vi "Cowl.vi"() -> ()   [LabVIEW 2019]
uses:
  outputs.vi
panel:
  out "Numeric":dbl
  in  "Desired_State 3":string
  in  "Desired_State 2":string
  in  "Desired_State":string
  in  "Current_State":string
  in  "Boolean":bool
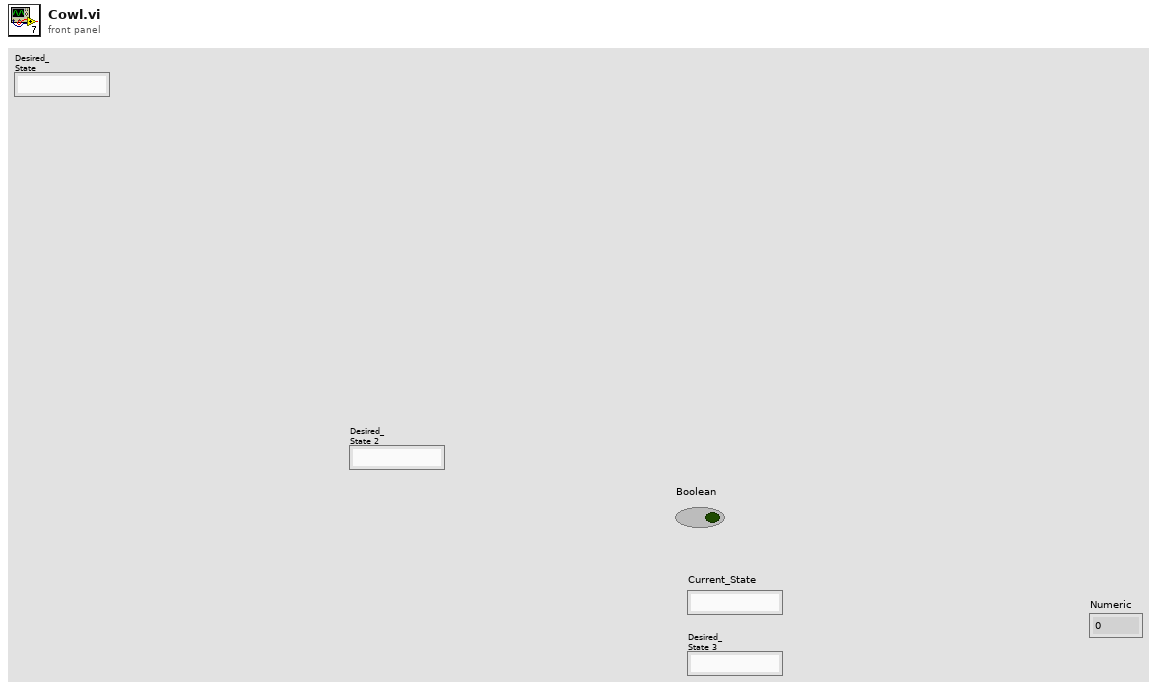
[diagram p1: front panel]
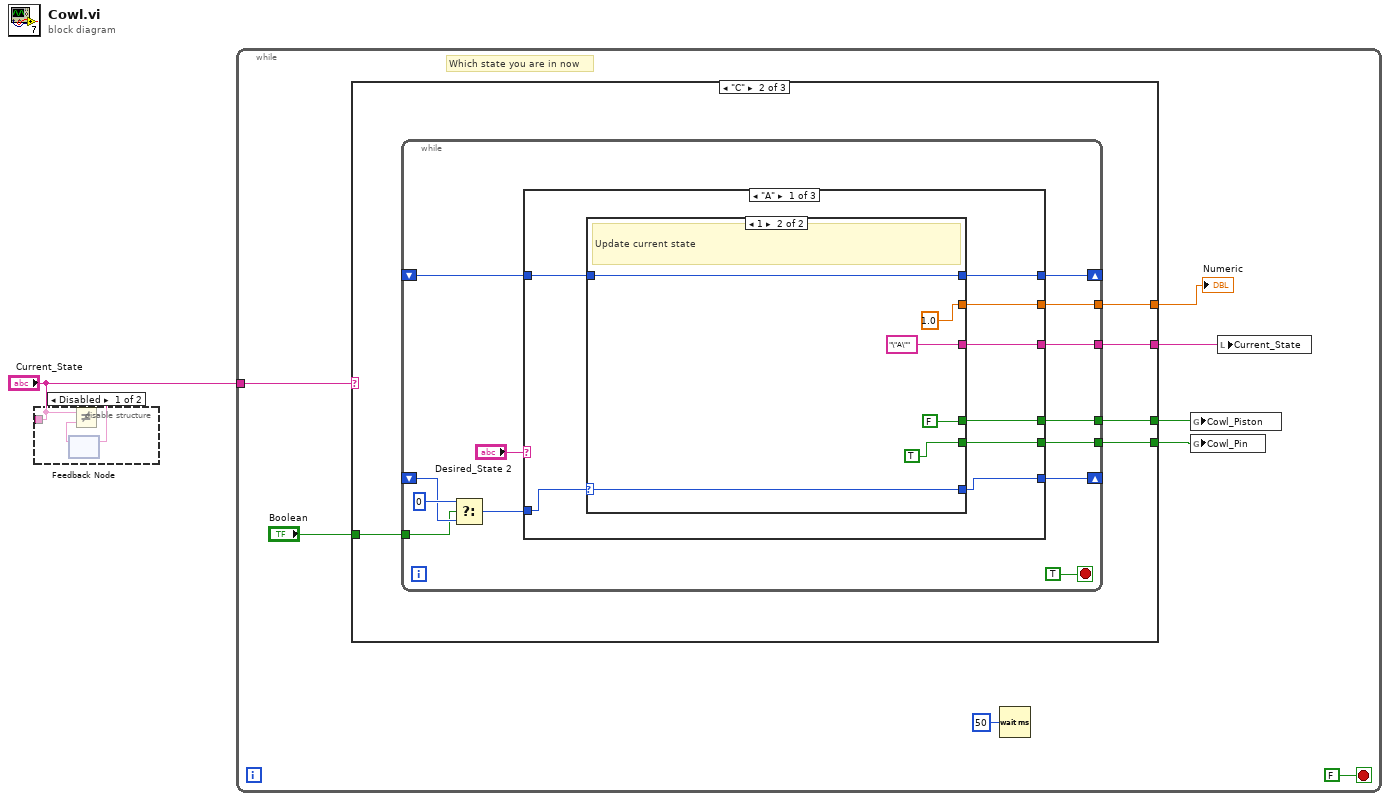
[diagram p0: block diagram]
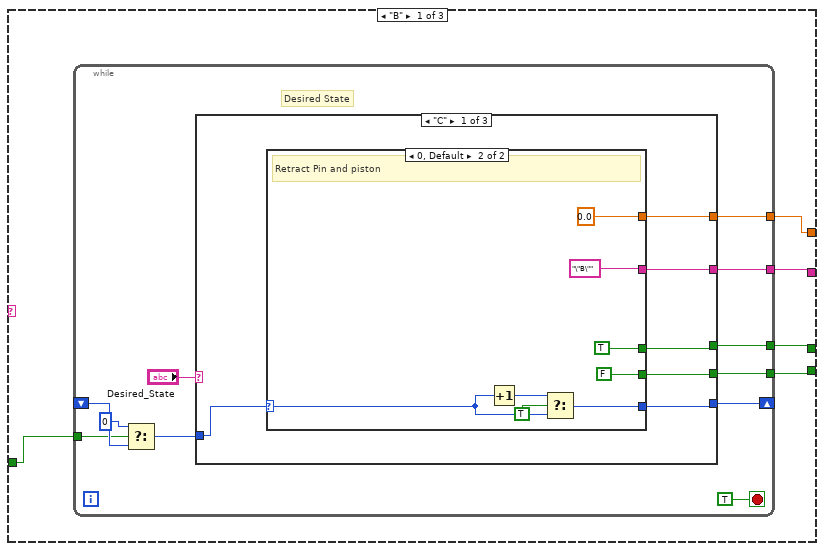
[diagram p3: hidden frame]
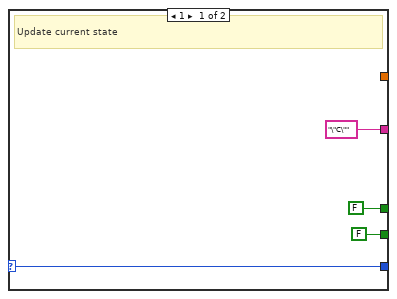
[diagram p4: hidden frame]
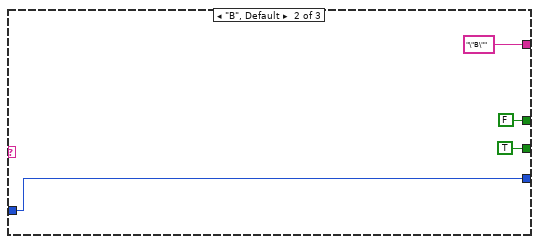
[diagram p5: hidden frame]
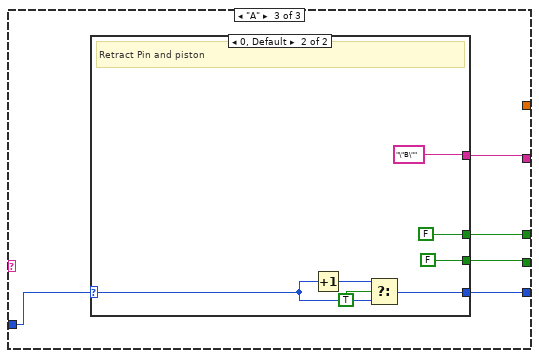
[diagram p6: hidden frame]
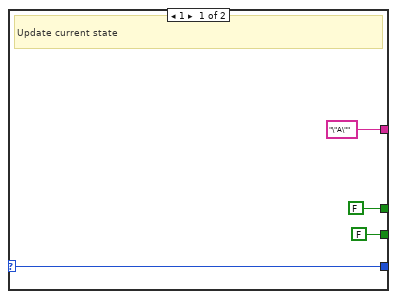
[diagram p7: hidden frame]
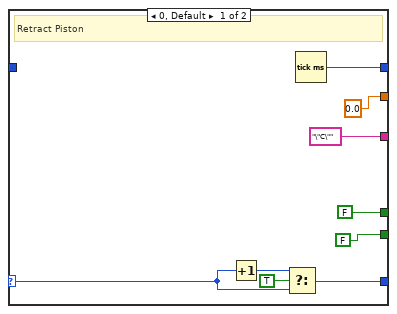
[diagram p8: hidden frame]
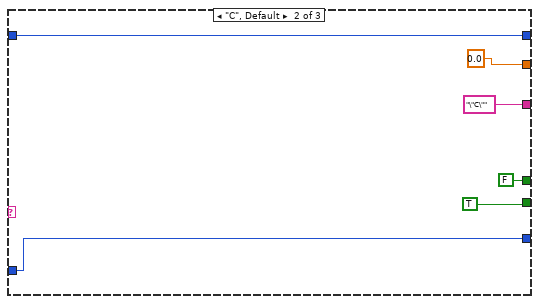
[diagram p9: hidden frame]
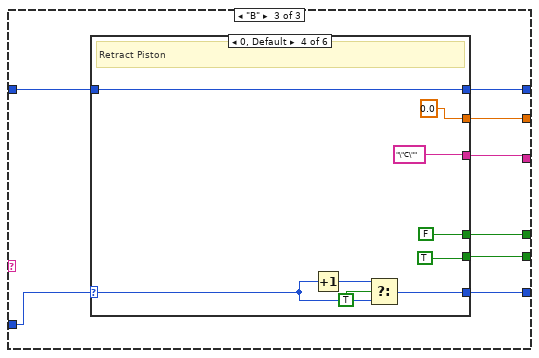
[diagram p10: hidden frame]
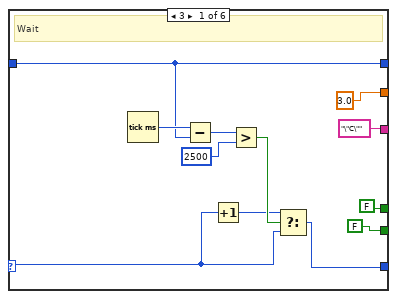
[diagram p11: hidden frame]
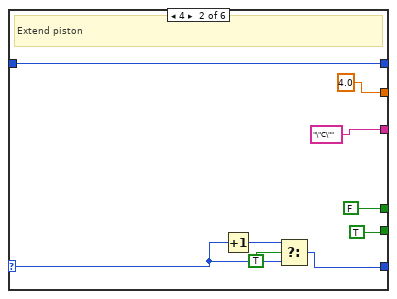
[diagram p12: hidden frame]
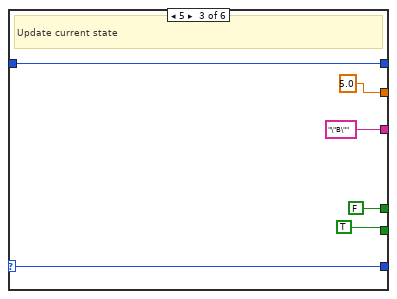
[diagram p13: hidden frame]
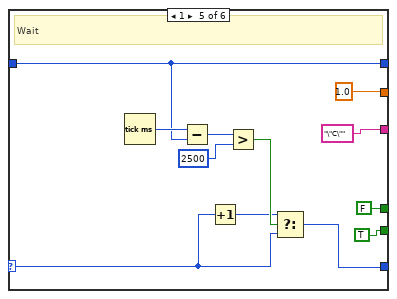
[diagram p14: hidden frame]
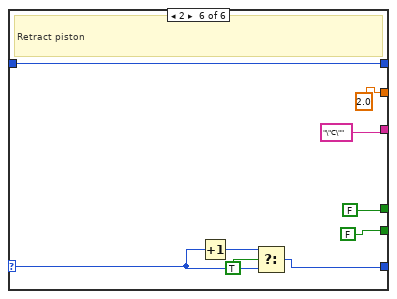
[diagram p15: hidden frame]
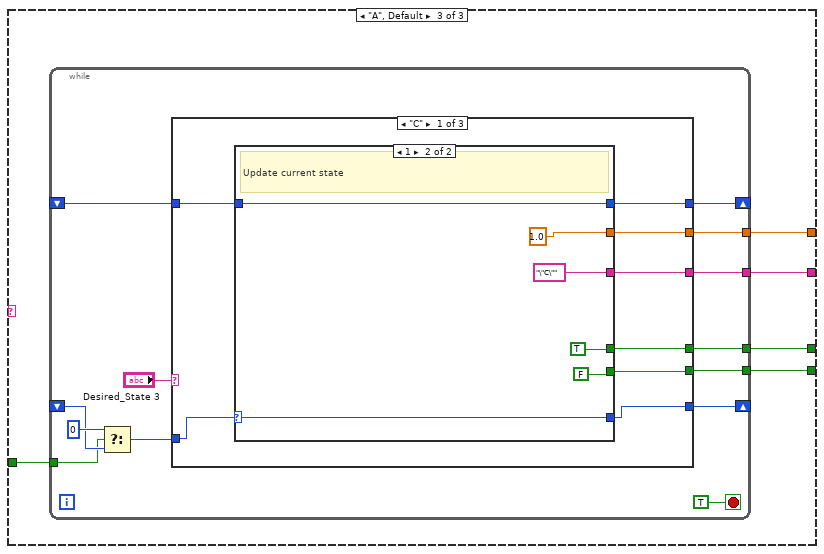
[diagram p16: hidden frame]
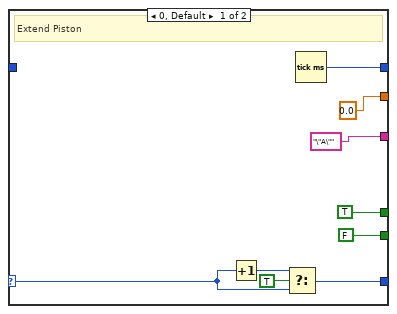
[diagram p17: hidden frame]
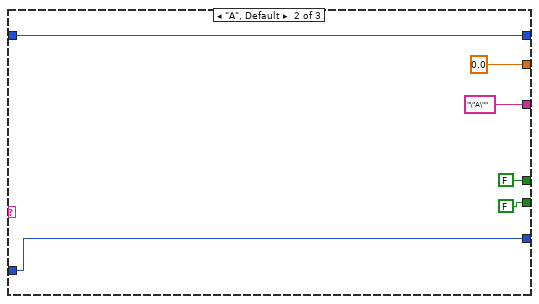
[diagram p18: hidden frame]
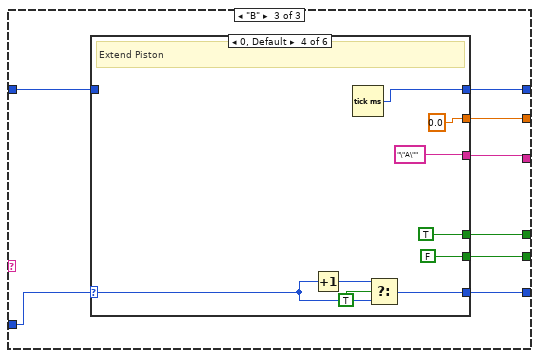
[diagram p19: hidden frame]
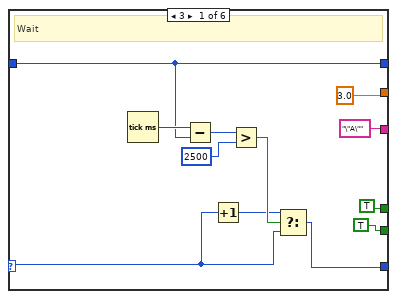
[diagram p20: hidden frame]
diagram:
  n1 = disable-structure shown="Disabled" {
    disable-tunnel: "Current_State" -> [w4 _]
    frame Disabled {
      n2 = feedback #1() -> (w3:string)  [unwired: 1 in]
      n3 = feedback-in #1(w4) -> ()
      n4 = Not Equal?(x=w4, y=w3) -> (x != y?=w2:bool)
    }
    frame Enabled {
    }
  }
  n5 = while {
    tunnel: "Current_State" -> [w12]
    stop <- FALSE stop-if-true
    # "Which state you are in now"
    n6 = case shown="\"C\"" w12 {
      tunnel: [w15 w70 w183] -> w9
      tunnel: [w16 w71 w182] -> w11
      tunnel: [w17 w69 w181] -> w10
      tunnel: [w14 w68 w180] -> w8
      tunnel: "Boolean" -> [w13 w67 w179]
      frame "B" {
        n7 = while {
          shift-right: [w24] -> _
          shift-left: _ -> [w26]
          tunnel: [w22] -> w15
          tunnel: [w21] -> w16
          tunnel: [w20] -> w17
          tunnel: [w19] -> w14
          tunnel: w13 -> [w18]
          stop <- TRUE stop-if-true
          # "Desired State"
          n8 = Select(t=0, s=w18, f=w26) -> (s? t:f=w25:i32)
          n9 = case shown="\"C\"" "Desired_State" {
            tunnel: w25 -> [w30 w50 w54]
            tunnel: [w31 w50 w55] -> w24
            tunnel: [w33 FALSE w53] -> w22
            tunnel: [w34 "\"B\"" w52] -> w21
            tunnel: [w32 TRUE w51] -> w20
            tunnel: [w29 _ _] -> w19
            frame "C" {
              n10 = case shown="0, Default" w30 {
                selector: w30 -> [w38 w46]
                tunnel: [w38 w45] -> w31
                tunnel: [FALSE TRUE] -> w33
                tunnel: ["\"C\"" "\"B\""] -> w34
                tunnel: [FALSE FALSE] -> w32
                tunnel: [_ 0.0 ("Numeric")] -> w29
                frame 1 {
                  # "Update current state"
                }
                frame 0, Default {
                  # "Retract Pin and piston"
                  n11 = Increment(x=w46) -> (x+1=w44:i32)
                  n12 = Select(t=w44, s=TRUE, f=w46) -> (s? t:f=w45:i32)
                }
              }
            }
            frame "B", Default {
            }
            frame "A" {
              n13 = case shown="0, Default" w54 {
                selector: w54 -> [w59 w66]
                tunnel: [w59 w65] -> w55
                tunnel: [FALSE FALSE] -> w53
                tunnel: ["\"A\"" "\"B\""] -> w52
                tunnel: [FALSE FALSE] -> w51
                frame 1 {
                  # "Update current state"
                }
                frame 0, Default {
                  # "Retract Pin and piston"
                  n14 = Increment(x=w66) -> (x+1=w64:i32)
                  n15 = Select(t=w64, s=TRUE, f=w66) -> (s? t:f=w65:i32)
                }
              }
            }
          }
        }
      }
      frame "C" {
        n16 = while {
          shift-right: [w82] -> _
          shift-left: _ -> [w83]
          shift-right: [w78] -> _
          shift-left: _ -> [w80]
          tunnel: [w76] -> w70
          tunnel: [w75] -> w71
          tunnel: [w74] -> w69
          tunnel: [w73] -> w68
          tunnel: w67 -> [w72]
          stop <- TRUE stop-if-true
          n17 = Select(t=0, s=w72, f=w80) -> (s? t:f=w79:i32)
          n18 = case shown="\"A\"" "Desired_State 2" {
            tunnel: w83 -> [w87 w113 w118]
            tunnel: [w90 w113 w117] -> w82
            tunnel: w79 -> [w92 w112 w120]
            tunnel: [w91 w112 w121] -> w78
            tunnel: [w89 FALSE w119] -> w76
            tunnel: [w88 "\"C\"" w116] -> w75
            tunnel: [w86 TRUE w115] -> w74
            tunnel: [w85 0.0 ("Numeric") w114] -> w73
            frame "A" {
              n19 = case shown="1" w92 {
                selector: w92 -> [w101 w107]
                tunnel: [w100 w107] -> w91
                tunnel: [FALSE FALSE] -> w89
                tunnel: [w96 w105] -> w90
                tunnel: ["\"C\"" "\"A\""] -> w88
                tunnel: w87 -> [_ w105]
                tunnel: [FALSE TRUE] -> w86
                tunnel: [0.0 ("Numeric") 1.0 ("Numeric")] -> w85
                frame 0, Default {
                  # "Retract Piston"
                  n20 = Increment(x=w101) -> (x+1=w99:i32)
                  n21 = Select(t=w99, s=TRUE, f=w101) -> (s? t:f=w100:i32)
                  n22 = Tick Count (ms)() -> (millisecond timer value=w96:u32)
                }
                frame 1 {
                  # "Update current state"
                }
              }
            }
            frame "C", Default {
            }
            frame "B" {
              n23 = case shown="0, Default" w120 {
                selector: w120 -> [w127 w138 w148 w157 w164 w174]
                tunnel: [w126 w139 w148 w156 w163 w173] -> w121
                tunnel: [FALSE FALSE FALSE FALSE FALSE FALSE] -> w119
                tunnel: w118 -> [w128 w137 w147 w153 w167 w178]
                tunnel: [w128 w137 w147 w153 w167 w178] -> w117
                tunnel: ["\"C\"" "\"C\"" "\"B\"" "\"C\"" "\"C\"" "\"C\""] -> w116
                tunnel: [FALSE TRUE TRUE TRUE TRUE FALSE] -> w115
                tunnel: [3.0 ("Numeric") 4.0 ("Numeric") 5.0 ("Numeric") 0.0 ("Numeric") 1.0 ("Numeric") 2.0 ("Numeric")] -> w114
                frame 3 {
                  # "Wait"
                  n24 = Tick Count (ms)() -> (millisecond timer value=w133:u32)
                  n25 = Subtract(x=w133, y=w128) -> (x-y=w132:u32)
                  n26 = Increment(x=w127) -> (x+1=w129:i32)
                  n27 = Greater?(x=w132, y=u32 2500) -> (0:w131:bool)
                  n28 = Select(t=w129, s=w131, f=w127) -> (s? t:f=w126:i32)
                }
                frame 4 {
                  # "Extend piston"
                  n29 = Increment(x=w138) -> (x+1=w141:i32)
                  n30 = Select(t=w141, s=TRUE, f=w138) -> (s? t:f=w139:i32)
                }
                frame 5 {
                  # "Update current state"
                }
                frame 0, Default {
                  # "Retract Piston"
                  n31 = Increment(x=w157) -> (x+1=w155:i32)
                  n32 = Select(t=w155, s=TRUE, f=w157) -> (s? t:f=w156:i32)
                }
                frame 1 {
                  # "Wait"
                  n33 = Tick Count (ms)() -> (millisecond timer value=w169:u32)
                  n34 = Subtract(x=w169, y=w167) -> (x-y=w168:u32)
                  n35 = Increment(x=w164) -> (x+1=w162:i32)
                  n36 = Greater?(x=w168, y=u32 2500) -> (0:w166:bool)
                  n37 = Select(t=w162, s=w166, f=w164) -> (s? t:f=w163:i32)
                }
                frame 2 {
                  # "Retract piston"
                  n38 = Increment(x=w174) -> (x+1=w176:i32)
                  n39 = Select(t=w176, s=TRUE, f=w174) -> (s? t:f=w173:i32)
                }
              }
            }
          }
        }
      }
      frame "A", Default {
        n40 = while {
          shift-right: [w194] -> _
          shift-left: _ -> [w195]
          shift-right: [w190] -> _
          shift-left: _ -> [w192]
          tunnel: [w188] -> w183
          tunnel: [w187] -> w182
          tunnel: [w186] -> w181
          tunnel: [w185] -> w180
          tunnel: w179 -> [w184]
          stop <- TRUE stop-if-true
          n41 = Select(t=0, s=w184, f=w192) -> (s? t:f=w191:i32)
          n42 = case shown="\"C\"" "Desired_State 3" {
            tunnel: w195 -> [w199 w225 w230]
            tunnel: [w202 w225 w229] -> w194
            tunnel: w191 -> [w204 w224 w232]
            tunnel: [w203 w224 w233] -> w190
            tunnel: [w201 FALSE w231] -> w188
            tunnel: [w200 "\"A\"" w228] -> w187
            tunnel: [w198 FALSE w227] -> w186
            tunnel: [w197 0.0 ("Numeric") w226] -> w185
            frame "C" {
              n43 = case shown="1" w204 {
                selector: w204 -> [w213 w219]
                tunnel: [w212 w219] -> w203
                tunnel: [TRUE TRUE] -> w201
                tunnel: [w208 w217] -> w202
                tunnel: ["\"A\"" "\"C\""] -> w200
                tunnel: w199 -> [_ w217]
                tunnel: [FALSE FALSE] -> w198
                tunnel: [0.0 ("Numeric") 1.0 ("Numeric")] -> w197
                frame 0, Default {
                  # "Extend Piston"
                  n44 = Increment(x=w213) -> (x+1=w211:i32)
                  n45 = Select(t=w211, s=TRUE, f=w213) -> (s? t:f=w212:i32)
                  n46 = Tick Count (ms)() -> (millisecond timer value=w208:u32)
                }
                frame 1 {
                  # "Update current state"
                }
              }
            }
            frame "A", Default {
            }
            frame "B" {
              n47 = case shown="0, Default" w232 {
                selector: w232 -> [w239 w250 w260 w269 w276 w286]
                tunnel: [w238 w251 w260 w268 w275 w285] -> w233
                tunnel: [TRUE FALSE FALSE TRUE TRUE TRUE] -> w231
                tunnel: w230 -> [w240 w249 w259 _ w279 w290]
                tunnel: [w240 w249 w259 w262 w279 w290] -> w229
                tunnel: ["\"A\"" "\"A\"" "\"B\"" "\"A\"" "\"A\"" "\"A\""] -> w228
                tunnel: [TRUE TRUE TRUE FALSE FALSE TRUE] -> w227
                tunnel: [3.0 ("Numeric") 4.0 ("Numeric") 5.0 ("Numeric") 0.0 ("Numeric") 1.0 ("Numeric") 2.0 ("Numeric")] -> w226
                frame 3 {
                  # "Wait"
                  n48 = Tick Count (ms)() -> (millisecond timer value=w245:u32)
                  n49 = Subtract(x=w245, y=w240) -> (x-y=w244:u32)
                  n50 = Increment(x=w239) -> (x+1=w241:i32)
                  n51 = Greater?(x=w244, y=u32 2500) -> (0:w243:bool)
                  n52 = Select(t=w241, s=w243, f=w239) -> (s? t:f=w238:i32)
                }
                frame 4 {
                  # "Retract piston"
                  n53 = Increment(x=w250) -> (x+1=w253:i32)
                  n54 = Select(t=w253, s=TRUE, f=w250) -> (s? t:f=w251:i32)
                }
                frame 5 {
                  # "Update current state"
                }
                frame 0, Default {
                  # "Extend Piston"
                  n55 = Increment(x=w269) -> (x+1=w267:i32)
                  n56 = Tick Count (ms)() -> (millisecond timer value=w262:u32)
                  n57 = Select(t=w267, s=TRUE, f=w269) -> (s? t:f=w268:i32)
                }
                frame 1 {
                  # "Wait"
                  n58 = Tick Count (ms)() -> (millisecond timer value=w281:u32)
                  n59 = Subtract(x=w281, y=w279) -> (x-y=w280:u32)
                  n60 = Increment(x=w276) -> (x+1=w274:i32)
                  n61 = Greater?(x=w280, y=u32 2500) -> (0:w278:bool)
                  n62 = Select(t=w274, s=w278, f=w276) -> (s? t:f=w275:i32)
                }
                frame 2 {
                  # "Extend piston"
                  n63 = Increment(x=w286) -> (x+1=w288:i32)
                  n64 = Select(t=w288, s=TRUE, f=w286) -> (s? t:f=w285:i32)
                }
              }
            }
          }
        }
      }
    }
    "Numeric" <- w8
    n65 = Wait (ms)(milliseconds to wait=u32 50) -> ()  [unwired: 1 out]
    n66 = global write "outputs.vi" "Cowl_Piston"(w9) -> ()
    n67 = global write "outputs.vi" "Cowl_Pin"(w10) -> ()
    n68 = local write "Current_State"(w11) -> ()
  }
